vi "OE1022D_Auto_Scale.vi"(0 "VISA resource name":refnum<visa-resource-name>, 1 "OE1022D A/B":u8(ring) items=["Channel A", "Channel B"], 5 "错误输入（无错误）":errorcluster) -> (14 "VISA resource name out":refnum<visa-resource-name>, 19 "错误输出":errorcluster)   [LabVIEW 2021]
doc: "Configures the reference source and the internal oscillator."
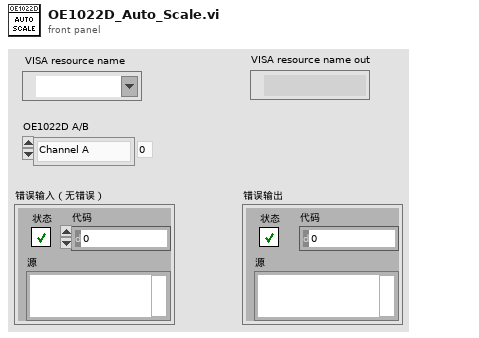
[diagram p1: front panel]
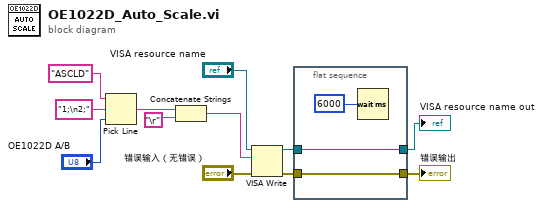
[diagram p0: block diagram]
diagram:
  n1 = Pick Line(string ("")="ASCLD", multi-line string="1;\n2;", line index="OE1022D A/B") -> (output string=w5:string)
  n2 = Concatenate Strings(w5, "\r") -> (w8:string)
  n3 = VISA Write(VISA resource name="VISA resource name", write buffer=w8, error in (no error)="错误输入（无错误）") -> (VISA resource name out=w4:refnum<visa-resource-name>, error out=w2:errorcluster)  [unwired: 1 out]
  n4 = flat-sequence {
    tunnel: [w14] -> w3
    tunnel: w4 -> [w14]
    tunnel: w2 -> [w13]
    tunnel: [w13] -> w1
    frame #0 {
      n5 = Wait (ms)(milliseconds to wait=u32 6000 ("等待时间（毫秒）")) -> ()  [unwired: 1 out]
    }
  }
  "VISA resource name out" <- w3
  "错误输出" <- w1
